vi "Write to Log File.vi"(3 "error in":errorcluster, 4 "HBDevRef":T1, 5 "Log Queue":refnum<queue>) -> (0 "error out":errorcluster, 1 "HBDevRef":T1, 2 "Log Queue":refnum<queue>)   [LabVIEW 2016]
uses:
  <vilib>/Rock Robotics/WPI/SerialPort/WPI_SerialPortRef.ctl
  Main/Robot Global Data.vi
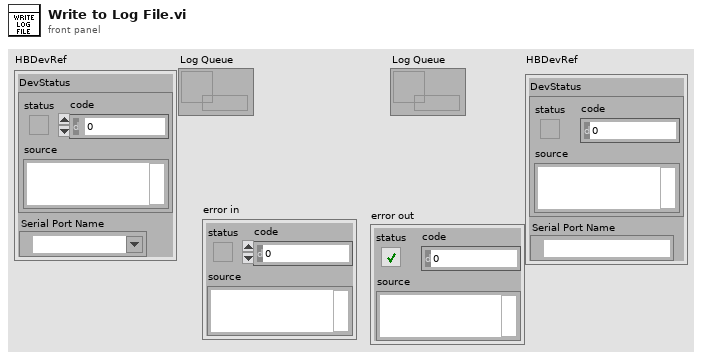
[diagram p1: front panel]
types:
  T1 = typedef "WPI_SerialPortRef.ctl" = cluster{"DevStatus":errorcluster, "Serial Port Name":refnum<visa-resource-name>}
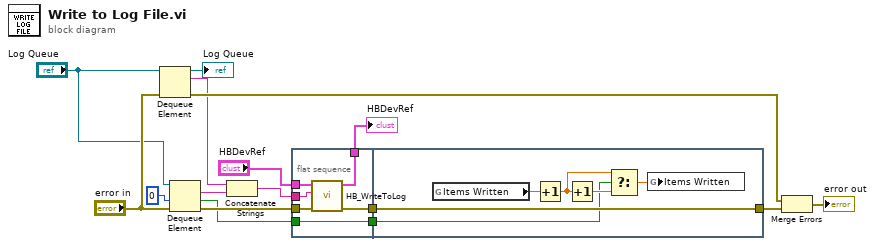
[diagram p0: block diagram]
diagram:
  n1 = Dequeue Element(queue="Log Queue", error in (no error)="error in") -> (queue out=→"Log Queue":refnum<queue>, element=w11:string, error out=w16:errorcluster)  [unwired: 1 in, 1 out]
  n2 = Dequeue Element(queue="Log Queue", timeout in ms (-1)=0, error in (no error)="error in") -> (element=w9:string, timed out?=w3:bool, error out=w7:errorcluster)  [unwired: 1 out]
  n3 = Concatenate Strings(w11, w9) -> (w10:string)
  n4 = flat-sequence {
    tunnel: [w22] -> w12
    tunnel: w10 -> [w21]
    tunnel: w7 -> [w20]
    tunnel: "HBDevRef" -> [w19]
    tunnel: [w18] -> w5
    tunnel: [w17] -> w4
    tunnel: w3 -> [w17]
    tunnel: [w28] -> w14
    tunnel: w12 -> [w28]
    tunnel: w4 -> [w23]
    frame #0 {
      n5 = call <vilib>:"HB_WriteToLog.vi"("error in (no error)"=w20, "Log string"=w21, "HBDevRef"=w19) -> ("error out"=w22:errorcluster, "HBDevRef"=w18:T1)  [unwired: 7 in]
    }
    frame #1 {
      n6 = global read "Robot Global Data.vi" "Items Written"() -> (w27:dbl)
      n7 = Increment(x=w27) -> (x+1=w26:dbl)
      n8 = Increment(x=w26) -> (x+1=w25:dbl)
      n9 = Select(t=w26, s=w23, f=w25) -> (s? t:f=w24:dbl)
      n10 = global write "Robot Global Data.vi" "Items Written"(w24) -> ()
    }
  }
  n11 = Merge Errors(w16, w14) -> (→"error out":errorcluster)
  "HBDevRef" <- w5
